vi "Render Window Setting.vi"(6 "Control Ref Queue":T1, 8 "error in (no error)":errorcluster, 11 "3D Plot.lvclass in":refnum<class "3D Plot.lvclass">) -> (0 "error out":errorcluster, 3 "3D Plot.lvclass out":refnum<class "3D Plot.lvclass">)   [LabVIEW 2017, in "3D Plot.lvclass"]
uses:
  <vilib>/Math Plots/3D Math Plots/3D Plot/3D Plot/3D Plot.lvclass
  <vilib>/Math Plots/3D Math Plots/3D Plot/Action String/3DMathPlot Ctrl Act Queue.ctl
  <vilib>/Math Plots/3D Math Plots/3D Plot/Action String/3DMathPlot Ctrl Act Cluster.ctl
  <vilib>/Math Plots/3D Math Plots/3D Plot/Action String/3DMathPlot State Class.ctl
  <vilib>/Math Plots/3D Math Plots/3D Plot/3D Plot/3D Plot.lvclass/3D Plot.ctl
  <vilib>/picture/3D Picture Control/NI_3D Picture Control.lvlib
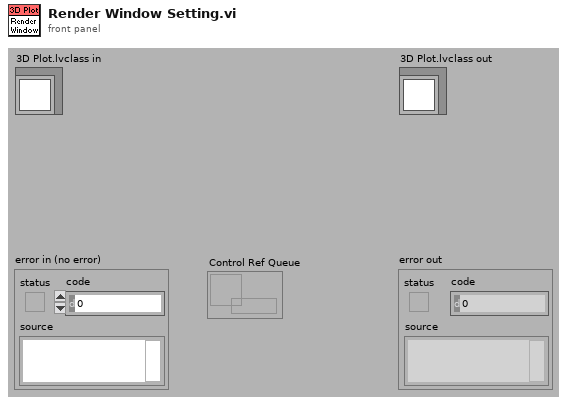
[diagram p1: front panel]
types:
  T1 = typedef "3DMathPlot Ctrl Act Queue.ctl" = refnum<queue>
  T2 = enum16{"None", "Spherical", "Flying", "Oriented"}
  T3 = enum32{"Towards X-Y Plane", "Towards X-Z Plane", "Towards Y-Z Plane", "User Defined"}
  T4 = cluster{"View Latitude":sgl, "View Longitude":sgl, "View Distance":sgl}
  T5 = typedef "3DMathPlot Ctrl Act Cluster.ctl" = cluster{"3D Picture Control":refnum<vi>, "Render Window Refnum":refnum<vi>, "XY Graph":refnum<vi>, "Intensity Graph":refnum<vi>, "Color Legend Palette":refnum<vi>, "Projection Palette":refnum<vi>, "XControl  Ref":refnum<vi>, "Facade Ref":refnum<vi>, "Export Image Ref":refnum<vi>, "Clear Data Flag":bool, "Display State Change Class":T6}
  T6 = typedef "3DMathPlot State Class.ctl" = enum16{"Update All Objects (Undo)", "Update Light Object Only", "Update Axis Object Only", "Update Plot Object Only", "Update Cursor Object Only", "Update Axis Plot Cursor Objects", "No Update"}
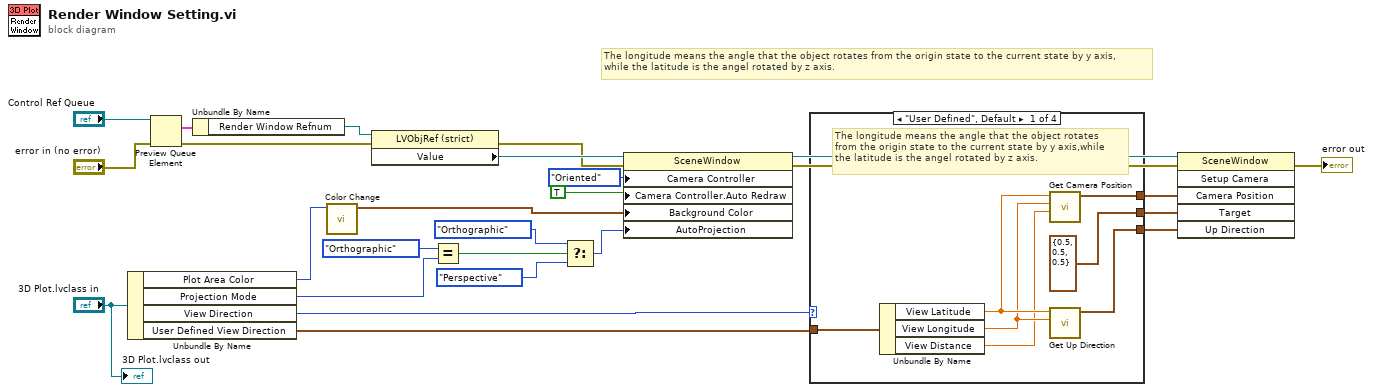
[diagram p0: block diagram]
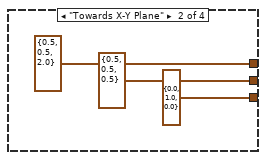
[diagram p2: hidden frame]
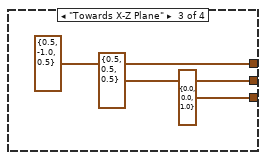
[diagram p3: hidden frame]
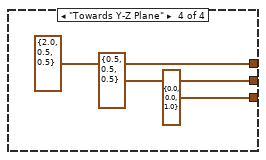
[diagram p4: hidden frame]
diagram:
  # "The longitude means the angle that the object rotates from the origin state to the current state by y axis,\nwhile the latitude is the angel rotated by z axis."
  n1 = Unbundle By Name("3D Plot.lvclass in") -> ("Plot Area Color"=w18:u32, "Projection Mode"=w3:enum16{"Orthographic", "Perspective"}, "View Direction"=w8:T3, "User Defined View Direction"=w4:T4)
  n2 = Preview Queue Element(queue="Control Ref Queue", error in (no error)="error in (no error)") -> (element=w14:T5, error out=w13:errorcluster)  [unwired: 3 out]
  n3 = Unbundle By Name(w14) -> ("Render Window Refnum"=w15:refnum<vi>)
  n4 = call <vilib>:"Color Change.vi"("Color"=w18) -> ("RGBA"=w12:cluster{"R":sgl, "G":sgl, "B":sgl, "A":sgl})  [unwired: 1 in, 9 out]
  n5 = property on="Property Node" class="LVObjRef (strict)"(reference=w15, error in=w13) -> (error out=w16:errorcluster, "Value"=w17:refnum<vi>)  [unwired: 1 out]
  n6 = Equal?(x=enum16{"Orthographic", "Perspective"}."Orthographic" ("y"), y=w3) -> (x = y?=w9:bool)
  n7 = Select(t=enum16{"None", "Perspective", "Orthographic"}."Orthographic" ("Automatic Projection Mode"), s=w9, f=enum16{"None", "Perspective", "Orthographic"}."Perspective" ("Automatic Projection Mode")) -> (s? t:f=w22:enum16{"None", "Perspective", "Orthographic"})
  n8 = property class="SceneWindow"(reference=w17, error in=w16, "Camera Controller"=T2."Oriented" ("Camera Controller:Type"), "Camera Controller.Auto Redraw"=TRUE ("Camera Controller:Auto Redraw"), "Background Color"=w12, "AutoProjection"=w22) -> (reference out=w2:refnum<vi>, error out=w1:errorcluster)
  n9 = case shown="\"User Defined\", Default" w8 {
    tunnel: [w33 cluster{"X":sgl, "Y":sgl, "Z":sgl} {"X"=0.5, "Y"=0.5, "Z"=2.0} ("Target") cluster{"X":sgl, "Y":sgl, "Z":sgl} {"X"=0.5, "Y"=-1.0, "Z"=0.5} ("Target") cluster{"X":sgl, "Y":sgl, "Z":sgl} {"X"=2.0, "Y"=0.5, "Z"=0.5} ("Target")] -> w7
    tunnel: [cluster{"X":sgl, "Y":sgl, "Z":sgl} {"X"=0.5, "Y"=0.5, "Z"=0.5} ("Target") cluster{"X":sgl, "Y":sgl, "Z":sgl} {"X"=0.5, "Y"=0.5, "Z"=0.5} ("Target") cluster{"X":sgl, "Y":sgl, "Z":sgl} {"X"=0.5, "Y"=0.5, "Z"=0.5} ("Target") cluster{"X":sgl, "Y":sgl, "Z":sgl} {"X"=0.5, "Y"=0.5, "Z"=0.5} ("Target")] -> w6
    tunnel: [w31 cluster{"X":sgl, "Y":sgl, "Z":sgl} {"X"=0.0, "Y"=1.0, "Z"=0.0} ("Target") cluster{"X":sgl, "Y":sgl, "Z":sgl} {"X"=0.0, "Y"=0.0, "Z"=1.0} ("Target") cluster{"X":sgl, "Y":sgl, "Z":sgl} {"X"=0.0, "Y"=0.0, "Z"=1.0} ("Target")] -> w5
    tunnel: w4 -> [w30 _ _ _]
    frame "User Defined", Default {
      # "The longitude means the angle that the object rotates \nfrom the origin state to the current state by y axis,while \nthe latitude is the angel rotated by z axis."
      n10 = Unbundle By Name(w30) -> ("View Latitude"=w29:sgl, "View Longitude"=w28:sgl, "View Distance"=w27:sgl)
      n11 = call <vilib>:"Get Camera Position.vi"("Distance"=w27, "Longitude"=w28, "Latitude"=w29) -> ("Camera Position"=w33:cluster{"X":sgl, "Y":sgl, "Z":sgl})  [unwired: 1 in, 7 out]
      n12 = call <vilib>:"Get Up Direction.vi"("Longitude"=w28, "Latitude"=w29) -> ("Up Direction"=w31:cluster{"X":sgl, "Y":sgl, "Z":sgl})  [unwired: 9 out]
    }
    frame "Towards X-Y Plane" {
    }
    frame "Towards X-Z Plane" {
    }
    frame "Towards Y-Z Plane" {
    }
  }
  n13 = invoke class="SceneWindow" method="Setup Camera"(reference=w2, error in=w1, "Camera Position"=w7, "Target"=w6, "Up Direction"=w5) -> (error out=→"error out":errorcluster)  [unwired: 1 in, 5 out]
  "3D Plot.lvclass out" <- "3D Plot.lvclass in"
